vi "UTIL_ResetDataStreams.vi"(6 "Results in":T1 {"Resistor 2" format="%.1f"; "Drain" format="%.3f"; "Resistor" format="%.1f"; "Fill" format="%.3f"}, 9 "TEST State Out":T4, 10 "Data in":dbl[][](array[numeric]), 11 "WaveformChart in":refnum<vi>) -> (1 "Value (Signaling)":bool, 2 "Results out":T1 {"Resistor 2" format="%.1f"; "Drain" format="%.3f"; "Resistor" format="%.1f"; "Fill" format="%.3f"}, 3 "Array":dbl[][](array[numeric]))   [LabVIEW 2024]
uses:
  Control Definitions/DEF_Results.ctl
  Control Definitions/DEF_ Results3.ctl
  Control Definitions/Def_ATPStatus.ctl
  Control Definitions/Def TestState.ctl
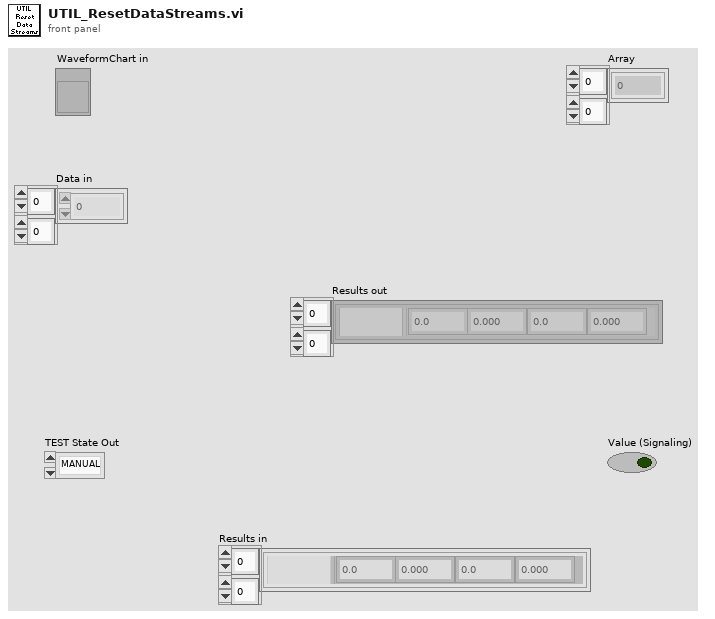
[diagram p1: front panel]
types:
  T1 = typedef "DEF_Results.ctl" = T2[][]
  T2 = typedef "DEF_ Results3.ctl" = cluster{"Fill":dbl, "Status":T3, "Resistor":dbl, "Drain":dbl, "Resistor 2":dbl}
  T3 = typedef "Def_ATPStatus.ctl" = i16
  T4 = typedef "Def TestState.ctl" = enum16{"MANUAL", "Start", "Pre-Fill", "Pre-Fill Measure", "Pre-Drain", "Pre-Drain Measure", "Init-Record", "Load Fill Spec", "Filling Hi", "Wait1", "Record Fill", "Load Drain Spec", "Draining Lo", "Wait2", "Record Drain", "Empty", "Done"}
  T5 = cluster{"ChA Ohms":dbl, "ChB Ohms":dbl, "Laser (raw)":dbl}[]
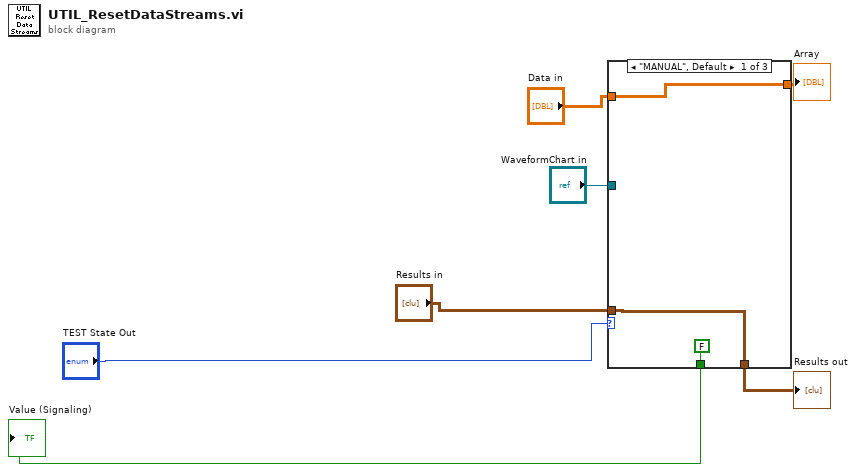
[diagram p0: block diagram]
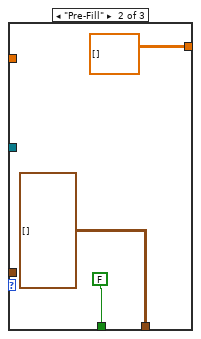
[diagram p2: hidden frame]
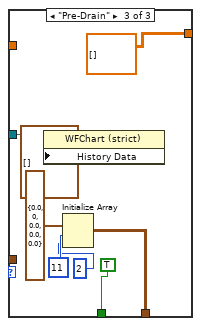
[diagram p3: hidden frame]
diagram:
  n1 = case shown="\"MANUAL\", Default" "TEST State Out" {
    tunnel: [w10 dbl[][] [] ("Array") dbl[][] [] ("Array")] -> w5
    tunnel: "Data in" -> [w10 _ _]
    tunnel: [w8 T1 [] ("Results in") w17] -> w1
    tunnel: [FALSE ("Value (Signaling)") FALSE ("Value (Signaling)") TRUE ("Value (Signaling)")] -> w6
    tunnel: "WaveformChart in" -> [_ _ w15]
    tunnel: "Results in" -> [w8 _ _]
    frame "MANUAL", Default {
    }
    frame "Pre-Fill" {
    }
    frame "Pre-Drain" {
      n2 = property on="Property Node" class="WFChart (strict)"(reference=w15, "History Data"=T5 []) -> ()  [unwired: 1 in, 2 out]
      n3 = Initialize Array(T2 {"Fill"=0.0, "Status"=0, "Resistor"=0.0, "Drain"=0.0, "Resistor 2"=0.0} ("Cluster 2"), 11 ("dimension size"), 2 ("dimension size")) -> (w17:T2[][])
    }
  }
  "Value (Signaling)" <- w6
  "Results out" <- w1
  "Array" <- w5
